vi "Mouse Write.vi"(3 "Timeout (ms)":i32=100, 4 "Write Data In":u8, 5 "Write Address":u8 format="%x", 6 "FPGA VI Reference In":refnum<k20>) -> (0 "Timed out?":bool, 2 "FPGA VI Reference Out":refnum<k20>)   [LabVIEW 2012]
uses:
  <vilib>/Utility/error.llb/Error Cluster From Error Code.vi
  <vilib>/rvi/errors/niLvFpgaAdjustHostInterfaceError.vi
  <vilib>/rvi/interface/nirviReadWriteControl/nirviReadWriteControl.xnode
  NiFpgaLv.dll
  <vilib>/rvi/interface/Simulation/niFpgaSimulationCallBeginRW.vi
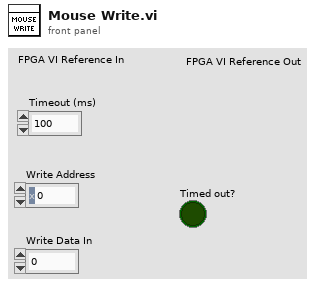
[diagram p1: front panel]
types:
  T1 = enum16{"idle", "set idle", "begin", "write", "read", "power down", "reset"}
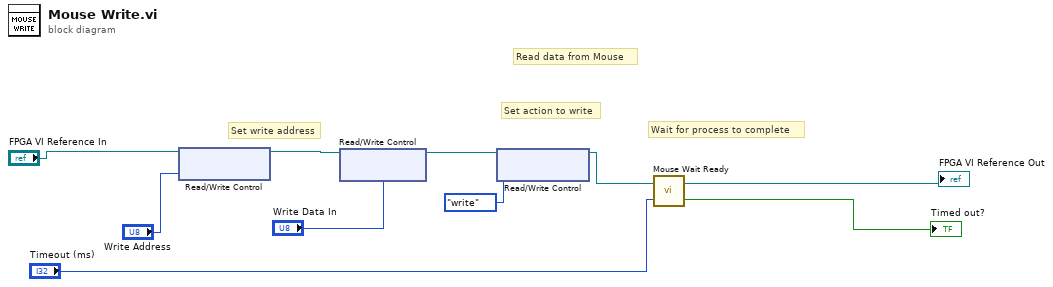
[diagram p0: block diagram]
diagram:
  # "Wait for process to complete"
  # "Set write address"
  # "Set action to write"
  # "Read data from Mouse"
  n1 = xnode "Read/Write Control"("FPGA VI Reference In"="FPGA VI Reference In", "Write Address"="Write Address") -> ("FPGA VI Reference Out"=w6:refnum<k20>)  [unwired: 1 in, 1 out]
  n2 = xnode "Read/Write Control"("FPGA VI Reference In"=w6, "Write Data In"="Write Data In") -> ("FPGA VI Reference Out"=w4:refnum<k20>)  [unwired: 1 in, 1 out]
  n3 = xnode "Read/Write Control"("FPGA VI Reference In"=w4, "Mouse Action"=T1."write") -> ("FPGA VI Reference Out"=w5:refnum<k20>)  [unwired: 1 in, 1 out]
  n4 = call "Mouse Wait Ready.vi"("Timeout (ms)"="Timeout (ms)", "Refnum in"=w5) -> ("Timeout"=→"Timed out?":bool, "Refnum out"=→"FPGA VI Reference Out":refnum<k20>)
